vi "Fit_plot_Gaussian.vi"(0 "X":ext[](array[numeric])=[-2.0, -1.0, 0.0, 1.0, 2.0, 3.0] format="%.2e", 5 "from":dbl format="%.2f", 7 "to":dbl format="%.2f", 9 "Y":ext[](array[numeric])=[17.0, 6.0, 1.0, 2.0, 9.0, 22.0] format="%.2e", 11 "DY":ext[](array[numeric])=[1.6999999999999999999, 0.59999999999999999997, 0.099999999999999999995, 0.19999999999999999999, 0.9, 2.1999999999999999998] format="%.2e") -> (2 "?":cluster{cluster{ext, ext}[]}[](graph)=[{[{-0.6097409095483231609, 1.9131742714567282e-25}, {-0.5942849916027894553, 1.5491733790203968e-25}, {-0.5788290736572557497, 1.2222526714426828e-25}, {-0.56337315571172204406, 9.324121487235825e-26}, {-0.54791723776618833847, 6.796518108630995e-26}, {-0.53246131982065463283, 4.6397165786123385e-26}, {-0.51700540187512092723, 2.853716897179855e-26}, {-0.5015494839295872216, 1.4385190643334717e-26}, {-0.486093565984053516, 3.94123080073335e-27}, {-0.4706376480385198104, -2.7947105560066505e-27}, {-0.45518173009298610479, -5.822633426884918e-27}, {-0.43972581214745239917, -5.1425378119018196e-27}, {-0.42426989420191869355, -7.544237110568042e-28}, {-0.40881397625638498793, 7.341708875649945e-27}, {-0.39335805831085128231, 1.9145859948218427e-26}, {-0.3779021403653175767, 3.465802950664864e-26}, {-0.36244622241978387107, 5.387821755094022e-26}, {-0.34699030447425016548, 7.680642408109335e-26}, {-0.33153438652871645986, 1.034426490971084e-25}, {-0.31607846858318275424, 1.3378689259898518e-25}]}, {[{-0.32099626065676166057, 3.1954140000000001329e-7}, {-0.33388985638954744083, 3.028025000000000126e-7}, {-0.34677198277837253924, 2.6036010000000001082e-7}, {-0.35964264437558956375, 2.1643890000000000901e-7}, {-0.37250184573240606217, 1.6418700000000000683e-7}, {-0.38534959139888473188, 1.4076750000000000585e-7}, {-0.39818588592394362971, 1.4076750000000000585e-7}, {-0.41101073385535638182, 1.6016000000000000666e-7}, {-0.42382413973975239334, 1.09008900000000004536e-7}, {-0.4366261081226170582, 9.6196100000000004e-8}, {-0.44941664354829196883, 4.8448400000000002014e-8}, {-0.46219575055997512585, 6.5088750000000002708e-8}, {-0.4749634336997211477, 6.7667600000000002816e-8}, {-0.48771969750844148023, 6.2562500000000002604e-8}, {-0.5004645465259046064, 9.009000000000000375e-8}, {-0.51319798529073625573, 1.1914230000000000496e-7}, {-0.52592001834041961396, 1.6016000000000000666e-7}, {-0.53863065021129553228, 1.8080350000000000752e-7}, {-0.55132988543856273724, 2.0722975000000000862e-7}, {-0.56401772855627803973, 2.7589800000000001147e-7}, {-0.5766941840973565447, 3.60360000000000015e-7}, {-0.58935925659357186053, 4.1643780000000001733e-7}, {-0.6020129505755563081, 4.3603560000000001814e-7}]}, {[{-0.32099626065676166057, 3.1890860000000001326e-7}, {-0.33388985638954744083, 3.0219750000000001257e-7}, {-0.34677198277837253924, 2.598399000000000108e-7}, {-0.35964264437558956375, 2.1601110000000000899e-7}, {-0.37250184573240606217, 1.6386300000000000681e-7}, {-0.38534959139888473188, 1.4048250000000000584e-7}, {-0.39818588592394362971, 1.4048250000000000584e-7}, {-0.41101073385535638182, 1.5984000000000000665e-7}, {-0.42382413973975239334, 1.08791100000000004523e-7}, {-0.4366261081226170582, 9.6003900000000003996e-8}, {-0.44941664354829196883, 4.835160000000000201e-8}, {-0.46219575055997512585, 6.4961250000000002702e-8}, {-0.4749634336997211477, 6.7532400000000002807e-8}, {-0.48771969750844148023, 6.2437500000000002596e-8}, {-0.5004645465259046064, 8.991000000000000374e-8}, {-0.51319798529073625573, 1.1890770000000000495e-7}, {-0.52592001834041961396, 1.5984000000000000665e-7}, {-0.53863065021129553228, 1.8044650000000000751e-7}, {-0.55132988543856273724, 2.068202500000000086e-7}, {-0.56401772855627803973, 2.7535200000000001144e-7}, {-0.5766941840973565447, 3.5964000000000001495e-7}, {-0.58935925659357186053, 4.1561220000000001728e-7}, {-0.6020129505755563081, 4.351644000000000181e-7}]}], 3 "sigma":dbl format="%.2f", 4 "delta sigma rms":dbl format="%.2f", 6 "m":dbl format="%.2f", 8 "delta m rms":dbl format="%.2f", 10 "A":dbl format="%.2f", 13 "Chi square":ext=5790999.8213589998395 format="%.3e", 14 "Degrees of freedom":ext=20.0 format="%.2f", 15 "delta A rms":dbl format="%.2f")   [LabVIEW 2014]
panel:
  # "Gaussian FIT"
  # "FS May,24 2000"
  # "DATA"
  # "Y = m0+m1*X+m2*X^2"
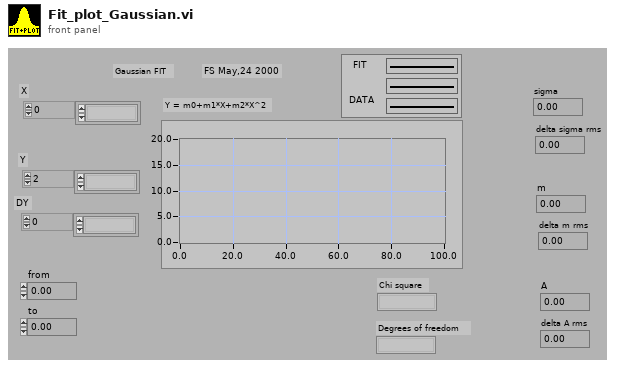
[diagram p1: front panel]
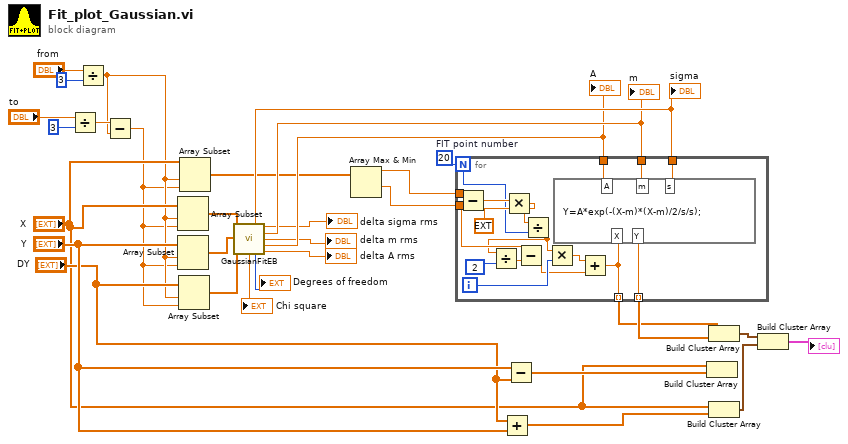
[diagram p0: block diagram]
diagram:
  w22 = 20  # FIT point number
  n1 = Divide(x="to", y=3) -> (x/y=w3:dbl)
  n2 = Divide(x="from", y=3) -> (x/y=w2:dbl)
  n3 = Subtract(x=w3, y=w2) -> (x-y=w1:dbl)
  n4 = Array Subset(array="X", index=w2, length=w1) -> (w14:ext[])
  n5 = Array Subset(array="Y", index=w2, length=w1) -> (w10:ext[])
  n6 = Array Subset(array="DY", index=w2, length=w1) -> (w8:ext[])
  n7 = Array Subset(array="X", index=w2, length=w1) -> (w6:ext[])
  n8 = call "GaussianFitEB.vi"("X"=w14, "Y"=w10, "DY"=w8) -> ("sigma"=w20:dbl, "delta sigma rms"=→"delta sigma rms":dbl, "m"=w19:dbl, "delta m rms"=→"delta m rms":dbl, "A"=w18:dbl, "Chi square"=→"Chi square":ext, "Degrees of freedom"=→"Degrees of freedom":i32, "delta A rms"=→"delta A rms":dbl)  [unwired: 5 in]
  "sigma" <- w20
  "m" <- w19
  "A" <- w18
  n9 = Array Max & Min(array=w6) -> (max value=w29:ext, min value=w28:ext)  [unwired: 2 out]
  n10 = for {
    N: w22 -> [w44]
    tunnel: w28 -> [w41]
    tunnel: w29 -> [w48]
    tunnel: [w36] -> w30 mode=indexing
    tunnel: [w49] -> w31 mode=indexing
    tunnel: w18 -> [w35]
    tunnel: w20 -> [w34]
    tunnel: w19 -> [w33]
    i -> [w42]
    n11 = Subtract(x=w48, y=w41) -> (x-y=w47:ext)
    n12 = Multiply(x=w47, y=ext 1.1) -> (x*y=w45:ext)
    n13 = Divide(x=w45, y=w44) -> (x/y=w37:ext)
    n14 = Divide(x=w37, y=2) -> (x/y=w38:ext)
    n15 = Subtract(x=w41, y=w38) -> (x-y=w40:ext)
    n16 = Multiply(x=w37, y=w42) -> (x*y=w43:ext)
    n17 = Add(x=w43, y=w40) -> (x+y=w36:ext)
    n18 = formula code="Y=A*exp(-(X-m)*(X-m)/2/s/s);"("X"=w36, "s"=w34, "m"=w33, "A"=w35) -> ("Y"=w49:dbl)
  }
  n19 = Add(x="DY", y="Y") -> (x+y=w26:ext[])
  n20 = Subtract(x="Y", y="DY") -> (x-y=w27:ext[])
  n21 = Build Cluster Array("X", w27) -> ()  [unwired: 1 out]
  n22 = Build Cluster Array(w30, w31) -> (w32:cluster{ext, "Y":dbl}[])
  n23 = Build Cluster Array("X", w26) -> (w24:cluster{ext, ext}[])
  n24 = Build Cluster Array(w32, w24) -> (→"?":cluster{cluster{ext, "Y":ext}[]}[])
